vi "OperacionesMatematicas.vi"() -> ()   [LabVIEW 2020]
panel:
  out "Sin(A-B)":dbl
  out "A-B":dbl
  out "A+B":dbl
  in  "B":dbl
  in  "A":dbl
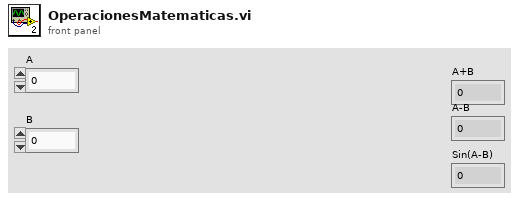
[diagram p1: front panel]
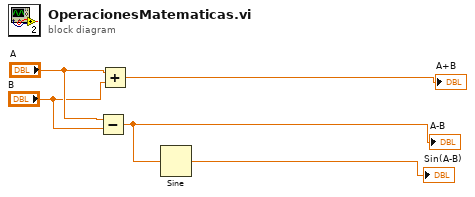
[diagram p0: block diagram]
diagram:
  n1 = Subtract(x="A", y="B") -> (x-y=w2:dbl)
  "A-B" <- w2
  n2 = Add(x="A", y="B") -> (x+y=→"A+B":dbl)
  n3 = Sine(x=w2) -> (sin(x)=→"Sin(A-B)":dbl)
